vi "Save_txtFile.vi"(4 "UseATI":bool, 5 "Data":string, 6 "DataCollect":bool, 7 "ForceMode":bool, 8 "UseVicon":bool, 11 "Filename":string) -> ()   [LabVIEW 2017]
uses:
  GlobalVariables.vi
panel:
  out "refnum out":refnum<file>
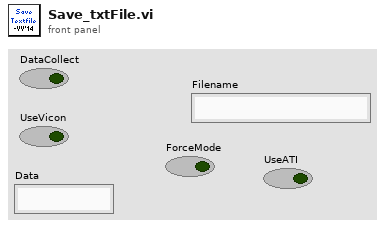
[diagram p1: front panel]
types:
  T1 = enum16{"open", "replace", "create", "open or create", "replace or create", "replace or create with confirmation"}
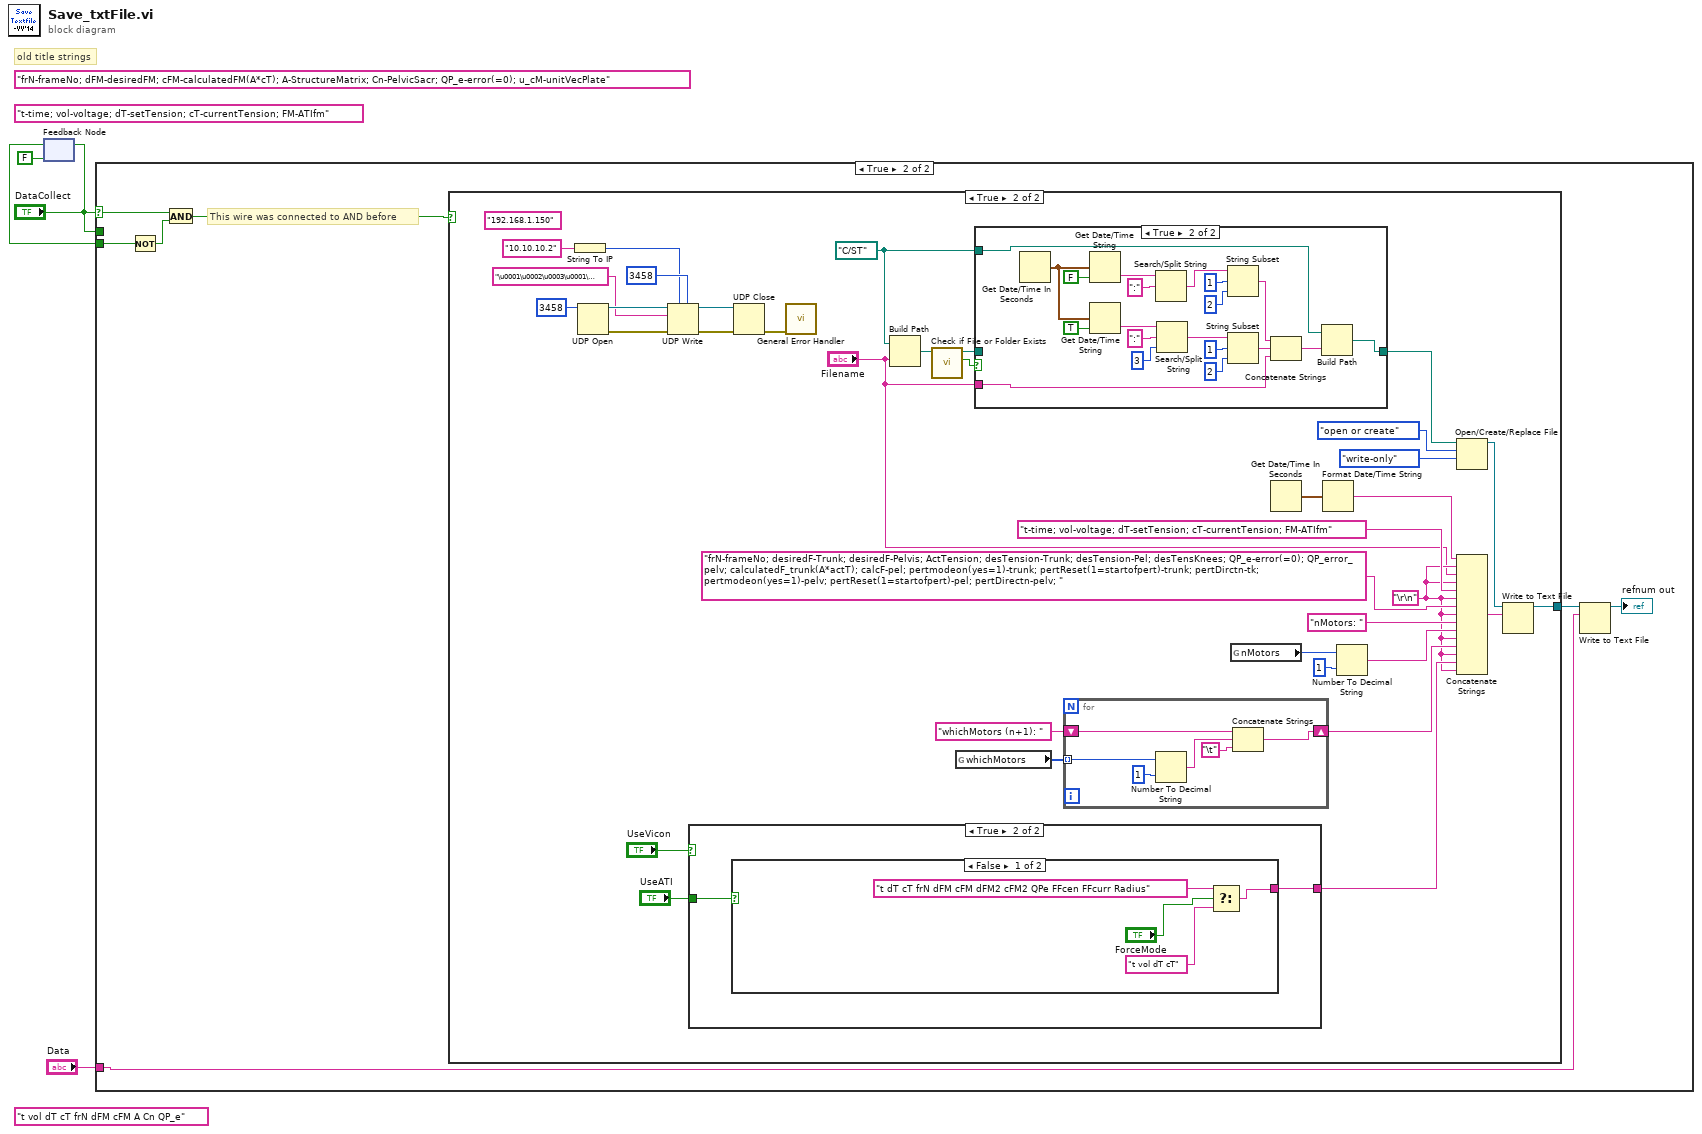
[diagram p0: block diagram]
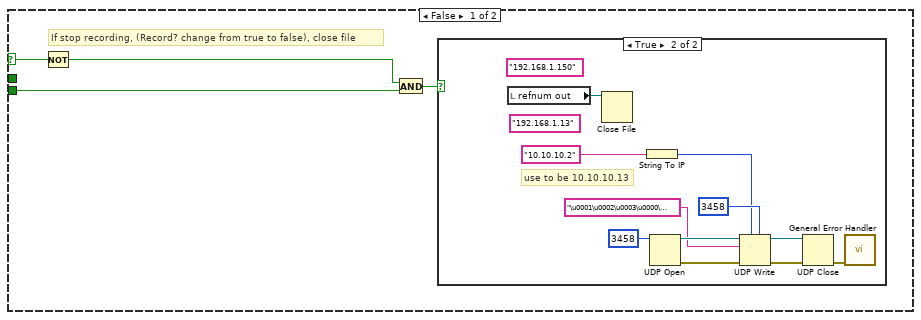
[diagram p2: hidden frame]
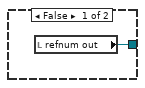
[diagram p4: hidden frame]
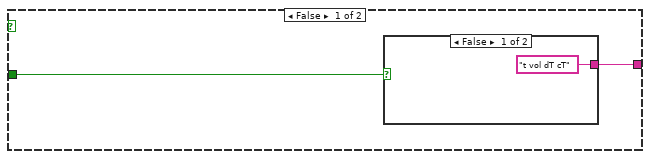
[diagram p6: hidden frame]
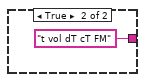
[diagram p7: hidden frame]
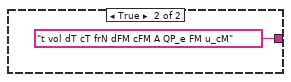
[diagram p8: hidden frame]
diagram:
  (unwired) "t vol dT cT frN dFM cFM A Cn QP_e"
  (unwired) "frN-frameNo; dFM-desiredFM; cFM-calculatedFM(A*cT); A-StructureMatrix; Cn-PelvicSacr; QP_e-error(=0); u_cM-unitVecPlate"
  (unwired) "t-time; vol-voltage; dT-setTension; cT-currentTension; FM-ATIfm"
  # "old title strings"
  n1 = feedback #1(FALSE) -> (w2:bool)
  n2 = feedback-in #1("DataCollect") -> ()
  n3 = case shown="True" "DataCollect" {
    selector: "DataCollect" -> [w7 w21]
    tunnel: "Data" -> [_ w25]
    tunnel: w2 -> [w6 w24]
    tunnel: "DataCollect" -> [_ _]
    frame False {
      # "If stop recording, (Record? change from true to false), close file"
      n4 = Not(x=w7) -> (.not. x?=w8:bool)
      n5 = And(x=w8, y=w6) -> (x .and. y?=w5:bool)
      n6 = case shown="True" w5 {
        frame False {
        }
        frame True {
          (unwired) "192.168.1.150" ("name")
          (unwired) "192.168.1.13" ("name")
          # "use to be 10.10.10.13"
          n7 = local read "refnum out"() -> (w19:refnum<file>)
          n8 = Close File(refnum=w19) -> ()  [unwired: 1 in, 2 out]
          n9 = String To IP(1:"10.10.10.2" ("name")) -> (0:w13:u32)
          n10 = UDP Open(11:u16 3458 ("port")) -> (port=w17:refnum<k16>, 0:w11:errorcluster)  [unwired: 4 in, 1 out]
          n11 = UDP Write(address=w13, port or service name=u16 3458, connection ID=w17, data in="\u0001\u0002\u0003\u0000\u0000\u0004\u0005\u0006", 8:w11) -> (error out=w12:errorcluster, 3:w16:refnum<k16>)  [unwired: 1 in]
          n12 = UDP Close(connection ID=w16, 8:w12) -> (error out=w18:errorcluster)  [unwired: 1 out]
          n13 = call <vilib>:"General Error Handler.vi"("error in (no error)"=w18) -> ()  [unwired: 10 in, 5 out]
        }
      }
    }
    frame True {
      # "This wire was connected to AND before"
      n14 = Not(x=w24) -> (.not. x?=w23:bool)
      n15 = And(x=w21, y=w23) -> (x .and. y?=w20:bool)
      n16 = case shown="True" w20 {
        tunnel: [w27 w63] -> w26
        frame False {
          n17 = local read "refnum out"() -> (w27:refnum<file>)
        }
        frame True {
          (unwired) "192.168.1.150" ("name")
          w38 = path "C:/ST" ("base path")
          w44 = "\r\n"
          n18 = String To IP(1:"10.10.10.2" ("name")) -> (0:w32:u32)
          n19 = UDP Open(11:u16 3458 ("port")) -> (port=w36:refnum<k16>, 0:w30:errorcluster)  [unwired: 4 in, 1 out]
          n20 = UDP Write(address=w32, port or service name=u16 3458, connection ID=w36, data in="\u0001\u0002\u0003\u0001\u0000\u0004\u0005\u0006", 8:w30) -> (error out=w31:errorcluster, 3:w35:refnum<k16>)  [unwired: 1 in]
          n21 = case shown="True" "UseVicon" {
            tunnel: [w92 w95] -> w45
            tunnel: "UseATI" -> [w91 w96]
            frame False {
              n22 = case shown="False" w91 {
                tunnel: ["t vol dT cT" "t vol dT cT FM"] -> w92
                frame False {
                }
                frame True {
                }
              }
            }
            frame True {
              n23 = case shown="False" w96 {
                tunnel: [w97 "t vol dT cT frN dFM cFM A QP_e FM u_cM"] -> w95
                frame False {
                  n24 = Select(t="t dT cT frN dFM cFM dFM2 cFM2 QPe FFcen FFcurr Radius", s="ForceMode", f="t vol dT cT") -> (s? t:f=w97:string)
                }
                frame True {
                }
              }
            }
          }
          n25 = UDP Close(connection ID=w35, 8:w31) -> (error out=w37:errorcluster)  [unwired: 1 out]
          n26 = call <vilib>:"General Error Handler.vi"("error in (no error)"=w37) -> ()  [unwired: 10 in, 5 out]
          n27 = Build Path(base path=w38, name or relative path="Filename") -> (appended path=w43:path)
          n28 = call <vilib>:"Check if File or Folder Exists.vi"("path"=w43) -> ("file or folder exists?"=w42:bool, "dup path"=w40:path)  [unwired: 8 in, 1 out]
          n29 = global read "GlobalVariables.vi" "whichMotors"() -> (w54:i32[])
          n30 = case shown="True" w42 {
            tunnel: "Filename" -> [_ w81]
            tunnel: w40 -> [w64 _]
            tunnel: [w64 w84] -> w39
            tunnel: w38 -> [_ w65]
            frame False {
            }
            frame True {
              n31 = Get Date/Time In Seconds() -> (seconds since 1Jan1904=w75:timestamp)
              n32 = Get Date/Time String(seconds (now)=w75, want seconds? (F)=FALSE) -> (time string=w80:string)  [unwired: 1 in, 1 out]
              n33 = Get Date/Time String(seconds (now)=w75, want seconds? (F)=TRUE) -> (time string=w73:string)  [unwired: 1 in, 1 out]
              n34 = Search/Split String(string=w80, search string/char (-)=":") -> (match + rest of string=w78:string)  [unwired: 1 in, 2 out]
              n35 = Search/Split String(string=w73, search string/char (-)=":", offset (0)=3) -> (match + rest of string=w68:string)  [unwired: 2 out]
              n36 = String Subset(string=w78, offset (0)=1, length (rest)=2 ("length (rest)")) -> (substring=w67:string)
              n37 = String Subset(string=w68, offset (0)=1, length (rest)=2 ("length (rest)")) -> (substring=w66:string)
              n38 = Concatenate Strings(w67, w66, w81) -> (w83:string)
              n39 = Build Path(base path=w65, name or relative path=w83) -> (appended path=w84:path)
            }
          }
          n40 = for {
            tunnel: w54 -> [w90] mode=indexing
            shift-right: [w85] -> w46
            shift-left: "whichMotors (n+1): " -> [w88]
            n41 = Number To Decimal String(number=w90, width (-)=i16 1) -> (decimal integer string=w87:string)
            n42 = Concatenate Strings(w88, w87, "\t") -> (w85:string)
          }
          n43 = global read "GlobalVariables.vi" "nMotors"() -> (w56:i32)
          n44 = Get Date/Time In Seconds() -> (seconds since 1Jan1904=w62:timestamp)
          n45 = Format Date/Time String(seconds (now)=w62) -> (date/time string=w61:string)  [unwired: 2 in]
          n46 = Number To Decimal String(number=w56, width (-)=i16 1) -> (decimal integer string=w47:string)
          n47 = Open/Create/Replace File(file path (use dialog)=w39, operation (0:open)=T1."open or create", access (0:read/write)=enum16{"read/write", "read-only", "write-only"}."write-only") -> (refnum out=w58:refnum<file>)  [unwired: 3 in, 2 out]
          n48 = Concatenate Strings(w61, w44, "Filename", w44, "t-time; vol-voltage; dT-setTension; cT-currentTension; FM-ATIfm", w44, "frN-frameNo; desiredF-Trunk; desiredF-Pelvis; ActTension; desTension-Trunk; desTension-Pel; desTensKnees; QP_e-error(=0); QP_error_pelv; calculatedF_trunk(A*actT); calcF-pel; pertmodeon(yes=1)-trunk; pertReset(1=startofpert)-trunk; pertDirctn-tk; pertmodeon(yes=1)-pelv; pertReset(1=startofpert)-pel; pertDirectn-pelv; ", w44, "nMotors: ", w47, w44, w46, w44, w45, w44) -> (w57:string)
          n49 = Write to Text File(file (use dialog)=w58, text=w57) -> (refnum out=w63:refnum<file>)  [unwired: 2 in, 2 out]
        }
      }
      n50 = Write to Text File(file (use dialog)=w26, text=w25) -> (refnum out=→"refnum out":refnum<file>)  [unwired: 2 in, 2 out]
    }
  }
